vi "NIFPGA-MCS.set bins per record.vi"(0 "i ref in":refnum<vi>, 2 "binsPerRecord":i32, 3 "ms timeout (10000)":i32=10000, 5 "error in (no error)":errorcluster) -> (14 "i ref out":refnum<vi>, 16 "binsPerRecord out":i32, 17 "timed out":bool, 19 "error out":errorcluster)   [LabVIEW 2014, in "NIFPGA-MCS.lvlib"]
doc: "Sets the number of bins in a spectrum of the MCS."
uses:
  NIFPGA-MCS.lvlib
  CSCore/CSApplicationBaseClasses/MCSBase/MCSBase.directionType.ctl
  CSCore/CSApplicationBaseClasses/MCSBase/MCSBase.serviceType.ctl
  CSlibraries/UtilityLib/UtilityLib.valueStatus.ctl
  CSCore/CSApplicationBaseClasses/DeviceBase/DeviceBase.lvlib
  CSCore/CSApplicationBaseClasses/MCSBase/MCSBase.lvlib
  CSlibraries/UtilityLib/UtilityLib.lvlib
  CSinstr.lib/NI-FPGA-MCS/host/instrumentDriver/NI-FPGA-MCS_Driver.lvlib
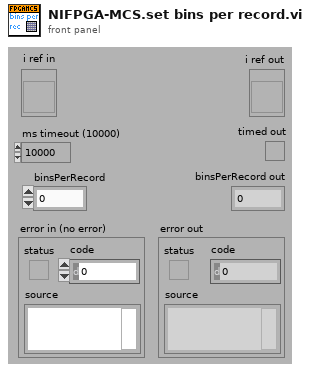
[diagram p1: front panel]
types:
  T1 = typedef "UtilityLib.lvlib/UtilityLib.valueStatus.ctl" = enum16{"no info available", "stand by/off", "on", "warning", "alarm/malfunction", "not implemented", "user action required", "important information", "system default", "control default", "indicator default", "button default"}
  T2 = typedef "MCSBase.lvlib/MCSBase.serviceType.ctl" = enum16{"counts", "totalCounts", "binWidth", "nOfBins", "nOfRecords", "status", "discrLevel", "discrSlope", "triggerLevel", "triggerSlope"}
  T3 = typedef "MCSBase.lvlib/MCSBase.directionType.ctl" = enum16{"unknown", "update actual value", "update nominal value", "update both"}
  T4 = typedef "NIFPGA-MCS.lvlib/NIFPGA-MCS.i attribute.ctl" = cluster{"fpgaViRef":T5}
  T5 = typedef "NI-FPGA-MCS_Driver.lvlib/fpga_vi_ref.ctl" = refnum<k20>
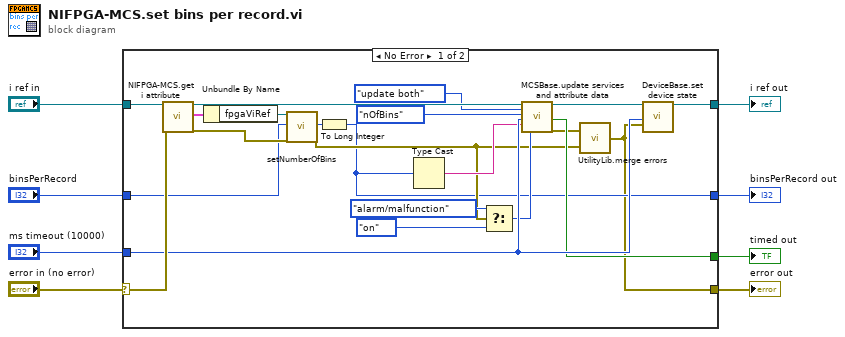
[diagram p0: block diagram]
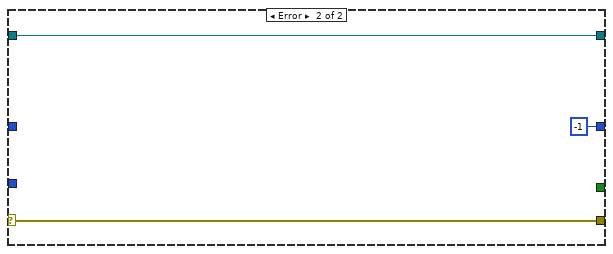
[diagram p2: hidden frame]
diagram:
  n1 = case shown="No Error" "error in (no error)" {
    selector: "error in (no error)" -> [w29 w32]
    tunnel: "i ref in" -> [w30 w33]
    tunnel: [w26 w33] -> w6
    tunnel: [w9 w32] -> w5
    tunnel: "ms timeout (10000)" -> [w22 _]
    tunnel: [w21 _] -> w3
    tunnel: "binsPerRecord" -> [w14 _]
    tunnel: [w10 -1] -> w1
    frame No Error {
      n2 = call "NIFPGA-MCS.get i attribute.vi"("i ref in"=w30, "error in (no error)"=w29) -> ("i ref out"=w24:refnum<vi>, "i attribute"=w27:T4, "error out"=w28:errorcluster)  [unwired: 15 in]
      n3 = Unbundle By Name(w27) -> ("fpgaViRef"=w25:T5)
      n4 = call "setNumberOfBins.vi"("fpga_vi_ref"=w25, "nOfBins (1024)"=w14, "error in (no error)"=w28) -> ("nOfBins out"=w11:u16, "error out"=w12:errorcluster)  [unwired: 14 in, 1 out]
      n5 = To Long Integer(number=w11) -> (32bit integer=w10:i32)
      n6 = Type Cast(x=w10) -> (*(type *) &x=w18:string)  [unwired: 1 in]
      n7 = Select(t=UtilityLib.valueStatus."alarm/malfunction", s=w12, f=UtilityLib.valueStatus."on" ("quality")) -> (s? t:f=w15:T1)
      n8 = call "MCSBase.update services and attribute data.vi"("i ref in"=w24, "direction"=MCSBase.directionType."update both", "service"=MCSBase.serviceType."nOfBins", "ms timeout (10000)"=w22, "value"=w18, "quality"=w15) -> ("i ref out"=w23:refnum<vi>, "timed out"=w21:bool, "error out"=w13:errorcluster)  [unwired: 11 in]
      n9 = call "UtilityLib.merge errors.vi"("error2 (no error)"=w12, "error1 (no error)"=w13) -> ("error out"=w9:errorcluster)
      n10 = call "DeviceBase.set device state.vi"("i ref in"=w23, "ms timeout (10000)"=w22, "device error"=w9) -> ("i ref out"=w26:refnum<vi>)  [unwired: 14 in, 2 out]
    }
    frame Error {
    }
  }
  "error out" <- w5
  "i ref out" <- w6
  "timed out" <- w3
  "binsPerRecord out" <- w1
